vi "Reset axes.vi"(8 "error in (no error)":errorcluster, 10 "Channel":T1="Z", 11 "Scientifica XYZ Gen1 in":refnum<class "Scientifica XYZ Gen1.lvclass">) -> (0 "error out":errorcluster, 3 "Scientifica XYZ Gen1 out":refnum<class "Scientifica XYZ Gen1.lvclass">)   [LabVIEW 2020, in "TranslationStageClassStructure.lvlib" / "Scientifica XYZ Gen1.lvclass"]
uses:
  Scientifica XYZ Gen1.lvclass
  Typedefs/XYZ channel ring.ctl
  Scientifica XYZ Gen1.lvclass/Scientifica XYZ Gen1.ctl
  Serial Comms/Serial Comms/Serial Comms.lvclass
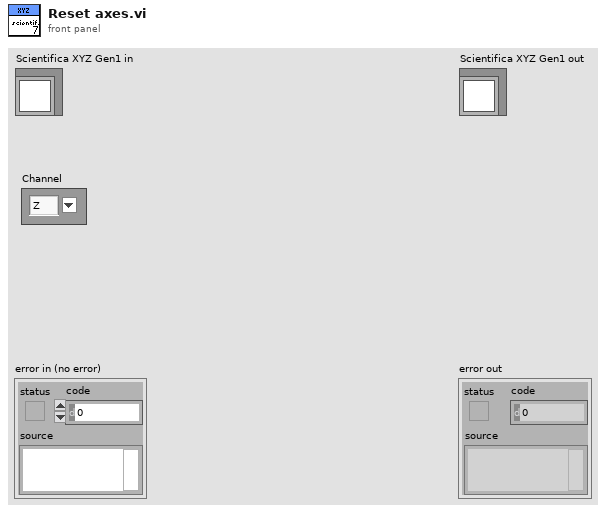
[diagram p1: front panel]
types:
  T1 = typedef "XYZ channel ring.ctl" = string
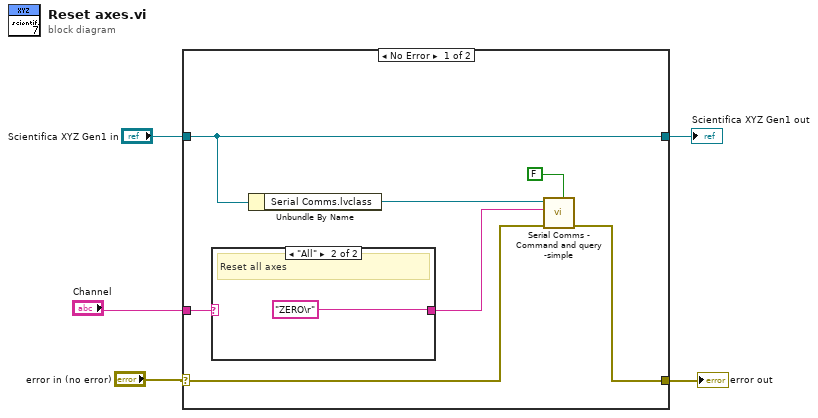
[diagram p0: block diagram]
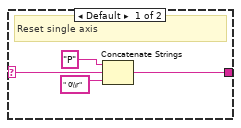
[diagram p2: hidden frame]
diagram:
  n1 = case shown="No Error" "error in (no error)" {
    selector: "error in (no error)" -> [w7 w18]
    tunnel: "Scientifica XYZ Gen1 in" -> [w11 w19]
    tunnel: [w11 w19] -> w3
    tunnel: "Channel" -> [w10 _]
    tunnel: [w6 w18] -> w1
    frame No Error {
      n2 = case shown="\"All\"" w10 {
        selector: w10 -> [w14 _]
        tunnel: [w13 "ZERO\r"] -> w8
        frame Default {
          # "Reset single axis"
          n3 = Concatenate Strings("P" ("string to write"), w14, " 0\\r" ("string")) -> (w13:string)
        }
        frame "All" {
          # "Reset all axes"
        }
      }
      n4 = Unbundle By Name(w11) -> ("Serial Comms.lvclass"=w12:refnum<class "Serial Comms.lvclass">)
      n5 = call "Serial Comms - Command and query -simple.vi"("Read response? (T)"=FALSE, "error in (no error)"=w7, "string to write"=w8, "Serial Comms in"=w12) -> ("error out"=w6:errorcluster)  [unwired: 3 in, 4 out]
    }
    frame Error {
    }
  }
  "error out" <- w1
  "Scientifica XYZ Gen1 out" <- w3
